vi "mod_Calculate Correction(Cont Zoom FFT).vi"(8 "error in (no error)":errorcluster, 9 "units":T3(ring)=enum."Watts", 10 "actual spectrum settings":T1={"center frequency"=-inf, "span"=-1.0, "resolution bandwidth"=-1.0, "window"=8, "spectral lines"=400, "%overlap"=0.0} {"%overlap" min=0.0 max=100.0 format="%.2f"; "window" items=["None ", "Hanning", "Hamming", "Blackman-Harris", "Exact Blackman", "Blackman", "Flat Top", "4 Term B-Harris ", "7 Term B-Harris", "Low Sidelobe"]; "resolution bandwidth" format="%.2p"; "center frequency" format="%.2p"; "span" format="%.2p"}, 11 "calibration array":T4(array[cluster]) {"array" format="%.2p"; "f2" format="%.2f"; "f1" format="%.2f"}) -> (0 "error out":errorcluster, 3 "correction":T2 {"spectrum correction"."correction factors" format="%.2f"; "spectrum correction"."df" format="%.2f"; "spectrum correction"."fo" format="%.2f"})   [LabVIEW 2020, in "niAMT.lvlib"]
doc: "Calculates a correction to compensate a spectrum for the amplitude response of signal conditioners and digitizers. Use your instrument drivers to determine the values you enter in the <B>calibration</B> cluster."
uses:
  <vilib>/addons/Modulation/niAMT.lvlib
  <vilib>/measure/masml.llb/ma_sml_CZ Spectrum Settings.ctl
  <vilib>/Analysis/1siggen.llb/Ramp Pattern by Samples.vi
  <vilib>/Analysis/NI_AALPro.lvlib
  <vilib>/Analysis/NI_AALBase.lvlib
  <vilib>/measure/NI_MAPro.lvlib
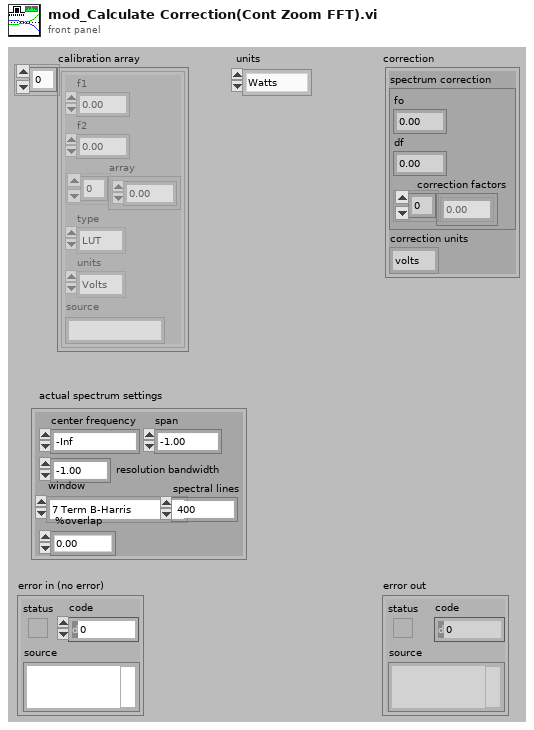
[diagram p1: front panel]
types:
  T1 = typedef "NI_MAPro.lvlib/ma_sml_CZ Spectrum Settings.ctl" = cluster{"center frequency":dbl, "span":dbl, "resolution bandwidth":dbl, "window":u16, "spectral lines":i32, "%overlap":dbl}
  T2 = cluster{"spectrum correction":cluster{"fo":dbl, "df":dbl, "correction factors":dbl[]}, "correction units":enum16{"volts", "watts", "dB"}}
  T3 = enum16{"Volts", "Watts", "dBm", "dBW", "dBV", "dBmV", "dBuV"}
  T4 = cluster{"f1":dbl, "f2":dbl, "array":sgl[], "type":enum16{"LUT", "polynomial"}, "units":enum16{"Volts", "Watts", "dBm", "dBW", "dBV", "dBmV", "dBuV"}, "source":string}[]
  T5 = cluster{cluster{dbl, dbl, dbl[]}, "correction units":enum16{"volts", "watts", "dB"}}
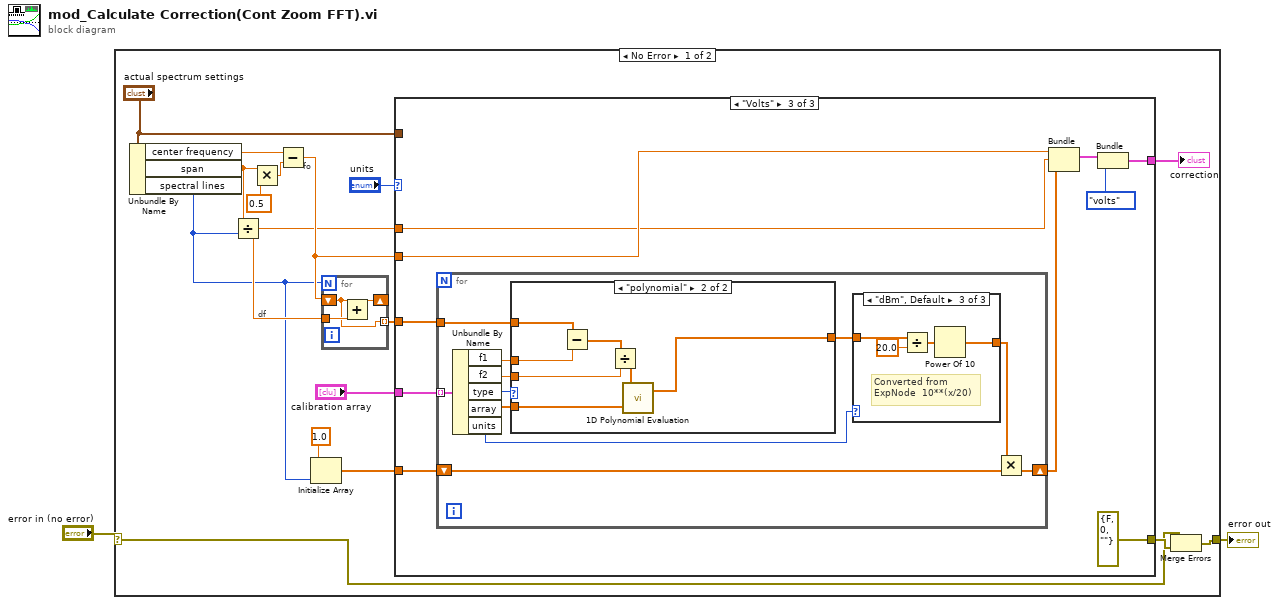
[diagram p0: block diagram]
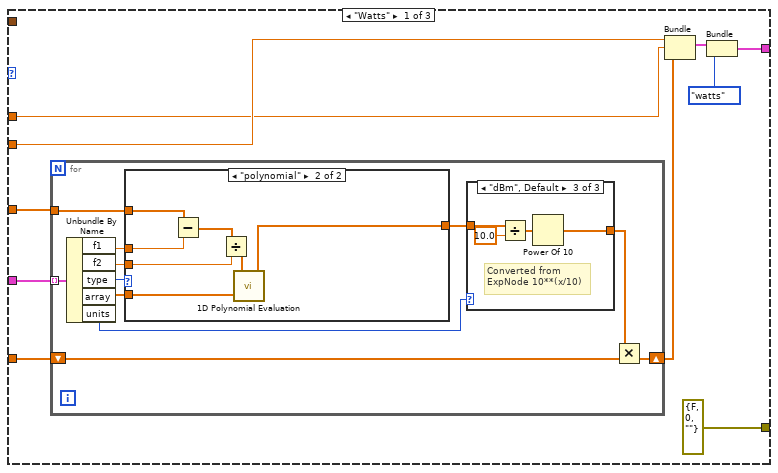
[diagram p2: hidden frame]
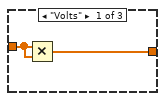
[diagram p3: hidden frame]
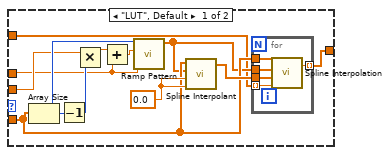
[diagram p5: hidden frame]
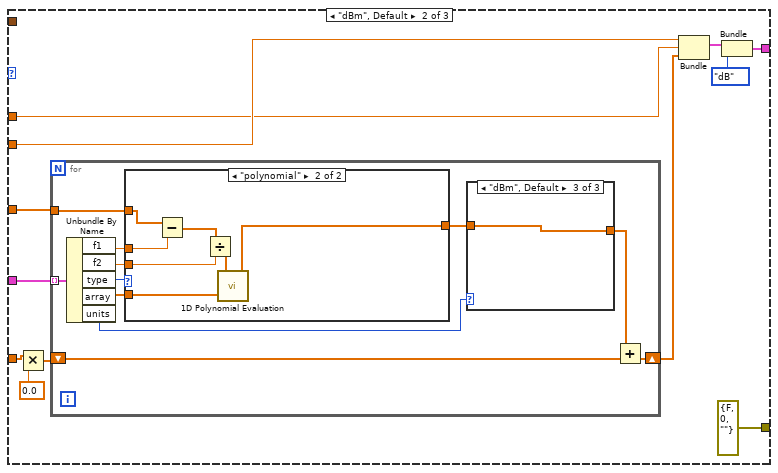
[diagram p6: hidden frame]
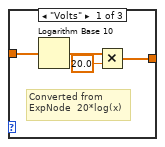
[diagram p7: hidden frame]
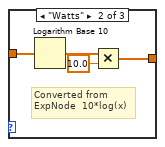
[diagram p8: hidden frame]
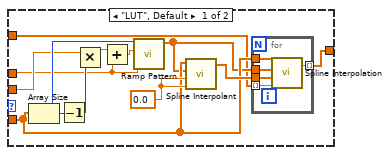
[diagram p9: hidden frame]
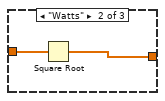
[diagram p11: hidden frame]
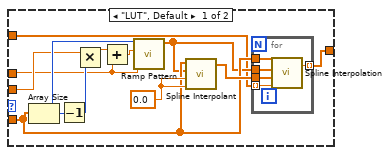
[diagram p12: hidden frame]
diagram:
  n1 = case shown="No Error" "error in (no error)" {
    selector: "error in (no error)" -> [w3 w183]
    tunnel: [w4 w183] -> w1
    frame No Error {
      # "df"
      # "fo"
      n2 = Unbundle By Name("actual spectrum settings") -> ("center frequency"=w15:dbl, "span"=w12:dbl, "spectral lines"=w7:i32)
      n3 = Divide(x=w12, y=w7) -> (x/y=w10:dbl)
      n4 = Multiply(x=w12, y=0.5) -> (x*y=w14:dbl)
      n5 = Subtract(x=w15, y=w14) -> (x-y=w11:dbl)
      n6 = Initialize Array(1.0, w7) -> (w17:dbl[])
      n7 = for {
        N: w7 -> [_]
        shift-right: [w181] -> _
        shift-left: w11 -> [w180]
        tunnel: w10 -> [w182]
        tunnel: [w180] -> w18 mode=indexing
        n8 = Add(x=w180, y=w182) -> (x+y=w181:dbl)
      }
      n9 = case shown="\"Volts\"" "units" {
        tunnel: "calibration array" -> [w29 w83 w137]
        tunnel: "actual spectrum settings" -> [_ _ _]
        tunnel: w18 -> [w28 w82 w136]
        tunnel: w17 -> [w26 w80 w134]
        tunnel: [errorcluster {"status"=FALSE, "code"=0, "source"=""} ("error IO") errorcluster {"status"=FALSE, "code"=0, "source"=""} ("error IO") errorcluster {"status"=FALSE, "code"=0, "source"=""} ("error IO")] -> w5
        tunnel: w11 -> [w25 w79 w133]
        tunnel: w10 -> [w24 w78 w132]
        tunnel: [w21 w75 w129] -> w8
        frame "Watts" {
          n10 = for {
            tunnel: w29 -> [w38] mode=indexing
            tunnel: w28 -> [w39]
            shift-right: [w30] -> w23
            shift-left: w26 -> [w32]
            n11 = Unbundle By Name(w38) -> ("f1"=w34:dbl, "f2"=w33:dbl, "type"=w40:enum16{"LUT", "polynomial"}, "array"=w37:sgl[], "units"=w36:T3)
            n12 = case shown="\"polynomial\"" w40 {
              tunnel: w39 -> [w49 w66]
              tunnel: w37 -> [w51 w68]
              tunnel: [w48 w65] -> w35
              tunnel: w34 -> [w53 w67]
              tunnel: w33 -> [w57 w69]
              frame "LUT", Default {
                w59 = 0.0 ("initial boundary")
                n13 = Array Size(array=w51) -> (size(s)=w58:i32)
                n14 = Decrement(x=w58) -> (x-1=w56:i32)
                n15 = Multiply(x=w57, y=w56) -> (x*y=w54:dbl)
                n16 = Add(x=w54, y=w53) -> (x+y=w55:dbl)
                n17 = call-poly <vilib>:"Ramp Pattern.vi"("start"=w53, "end"=w55, "samples"=w58) -> ("Ramp Pattern"=w50:dbl[])  [unwired: 7 in, 1 out]
                n18 = call <vilib>:"Spline Interpolant.vi"("final boundary"=w59, "initial boundary"=w59, "X"=w50, "Y"=w51) -> ("Interpolant"=w52:dbl[])  [unwired: 1 out]
                n19 = for {
                  tunnel: w52 -> [w64]
                  tunnel: w51 -> [w63]
                  tunnel: w50 -> [w62]
                  tunnel: w49 -> [w61] mode=indexing
                  tunnel: [w60] -> w48 mode=indexing
                  n20 = call <vilib>:"Spline Interpolation.vi"("x value"=w61, "Interpolant"=w64, "X"=w62, "Y"=w63) -> ("interpolation value"=w60:dbl)  [unwired: 1 out]
                }
              }
              frame "polynomial" {
                n21 = Subtract(x=w66, y=w67) -> (x-y=w71:dbl[])
                n22 = Divide(x=w71, y=w69) -> (x/y=w70:dbl[])
                n23 = call <vilib>:"1D Polynomial Evaluation.vi"("Coefficients: a"=w68, "X"=w70) -> ("Y"=w65:dbl[])  [unwired: 1 out]
              }
            }
            n24 = case shown="\"dBm\", Default" w36 {
              tunnel: w35 -> [w41 w43 w45]
              tunnel: [w42 w43 w44] -> w31
              frame "Volts" {
                n25 = Multiply(x=w41, y=w41) -> (x*y=w42:dbl[])
              }
              frame "Watts" {
              }
              frame "dBm", Default {
                # "Converted from\nExpNode 10**(x/10)"
                n26 = Divide(x=w45, y=10.0) -> (x/y=w47:dbl[])
                n27 = Power Of 10(x=w47) -> (10^x=w44:dbl[])
              }
            }
            n28 = Multiply(x=w31, y=w32) -> (x*y=w30:dbl[])
          }
          n29 = Bundle(w25, w24, w23) -> (w22:cluster{dbl, dbl, dbl[]})  [unwired: 1 out]
          n30 = Bundle(w22, "correction units"=enum16{"volts", "watts", "dB"}."watts") -> (w21:T5)  [unwired: 1 out]
        }
        frame "dBm", Default {
          n31 = Multiply(x=w80, y=0.0) -> (x*y=w74:dbl[])
          n32 = for {
            tunnel: w83 -> [w92] mode=indexing
            tunnel: w82 -> [w93]
            shift-right: [w84] -> w77
            shift-left: w74 -> [w86]
            n33 = Unbundle By Name(w92) -> ("f1"=w88:dbl, "f2"=w87:dbl, "type"=w94:enum16{"LUT", "polynomial"}, "array"=w91:sgl[], "units"=w90:T3)
            n34 = case shown="\"polynomial\"" w94 {
              tunnel: w93 -> [w105 w127]
              tunnel: w91 -> [w107 w126]
              tunnel: [w104 w125] -> w89
              tunnel: w88 -> [w109 w123]
              tunnel: w87 -> [w113 w121]
              frame "LUT", Default {
                w115 = 0.0 ("initial boundary")
                n35 = Array Size(array=w107) -> (size(s)=w114:i32)
                n36 = Decrement(x=w114) -> (x-1=w112:i32)
                n37 = Multiply(x=w113, y=w112) -> (x*y=w110:dbl)
                n38 = Add(x=w110, y=w109) -> (x+y=w111:dbl)
                n39 = call-poly <vilib>:"Ramp Pattern.vi"("start"=w109, "end"=w111, "samples"=w114) -> ("Ramp Pattern"=w106:dbl[])  [unwired: 7 in, 1 out]
                n40 = call <vilib>:"Spline Interpolant.vi"("final boundary"=w115, "initial boundary"=w115, "X"=w106, "Y"=w107) -> ("Interpolant"=w108:dbl[])  [unwired: 1 out]
                n41 = for {
                  tunnel: w108 -> [w120]
                  tunnel: w107 -> [w119]
                  tunnel: w106 -> [w118]
                  tunnel: w105 -> [w117] mode=indexing
                  tunnel: [w116] -> w104 mode=indexing
                  n42 = call <vilib>:"Spline Interpolation.vi"("x value"=w117, "Interpolant"=w120, "X"=w118, "Y"=w119) -> ("interpolation value"=w116:dbl)  [unwired: 1 out]
                }
              }
              frame "polynomial" {
                n43 = Subtract(x=w127, y=w123) -> (x-y=w124:dbl[])
                n44 = Divide(x=w124, y=w121) -> (x/y=w122:dbl[])
                n45 = call <vilib>:"1D Polynomial Evaluation.vi"("Coefficients: a"=w126, "X"=w122) -> ("Y"=w125:dbl[])  [unwired: 1 out]
              }
            }
            n46 = case shown="\"dBm\", Default" w90 {
              tunnel: w89 -> [w96 w100 w103]
              tunnel: [w95 w99 w103] -> w85
              frame "Volts" {
                # "Converted from\nExpNode \t20*log(x)"
                n47 = Logarithm Base 10(1:w96) -> (0:w97:dbl[])
                n48 = Multiply(x=w97, y=20.0) -> (x*y=w95:dbl[])
              }
              frame "Watts" {
                # "Converted from\nExpNode \t10*log(x)"
                n49 = Logarithm Base 10(1:w100) -> (0:w101:dbl[])
                n50 = Multiply(x=w101, y=10.0) -> (x*y=w99:dbl[])
              }
              frame "dBm", Default {
              }
            }
            n51 = Add(x=w85, y=w86) -> (x+y=w84:dbl[])
          }
          n52 = Bundle(w79, w78, w77) -> (w76:cluster{dbl, dbl, dbl[]})  [unwired: 1 out]
          n53 = Bundle(w76, "correction units"=enum16{"volts", "watts", "dB"}."dB") -> (w75:T5)  [unwired: 1 out]
        }
        frame "Volts" {
          n54 = for {
            tunnel: w137 -> [w146] mode=indexing
            tunnel: w136 -> [w147]
            shift-right: [w138] -> w131
            shift-left: w134 -> [w140]
            n55 = Unbundle By Name(w146) -> ("f1"=w142:dbl, "f2"=w141:dbl, "type"=w148:enum16{"LUT", "polynomial"}, "array"=w145:sgl[], "units"=w144:T3)
            n56 = case shown="\"polynomial\"" w148 {
              tunnel: w147 -> [w157 w174]
              tunnel: w145 -> [w159 w173]
              tunnel: [w156 w179] -> w143
              tunnel: w142 -> [w161 w175]
              tunnel: w141 -> [w165 w176]
              frame "LUT", Default {
                w167 = 0.0 ("initial boundary")
                n57 = Array Size(array=w159) -> (size(s)=w166:i32)
                n58 = Decrement(x=w166) -> (x-1=w164:i32)
                n59 = Multiply(x=w165, y=w164) -> (x*y=w162:dbl)
                n60 = Add(x=w162, y=w161) -> (x+y=w163:dbl)
                n61 = call-poly <vilib>:"Ramp Pattern.vi"("start"=w161, "end"=w163, "samples"=w166) -> ("Ramp Pattern"=w158:dbl[])  [unwired: 7 in, 1 out]
                n62 = call <vilib>:"Spline Interpolant.vi"("final boundary"=w167, "initial boundary"=w167, "X"=w158, "Y"=w159) -> ("Interpolant"=w160:dbl[])  [unwired: 1 out]
                n63 = for {
                  tunnel: w160 -> [w172]
                  tunnel: w159 -> [w171]
                  tunnel: w158 -> [w170]
                  tunnel: w157 -> [w169] mode=indexing
                  tunnel: [w168] -> w156 mode=indexing
                  n64 = call <vilib>:"Spline Interpolation.vi"("x value"=w169, "Interpolant"=w172, "X"=w170, "Y"=w171) -> ("interpolation value"=w168:dbl)  [unwired: 1 out]
                }
              }
              frame "polynomial" {
                n65 = Subtract(x=w174, y=w175) -> (x-y=w178:dbl[])
                n66 = Divide(x=w178, y=w176) -> (x/y=w177:dbl[])
                n67 = call <vilib>:"1D Polynomial Evaluation.vi"("Coefficients: a"=w173, "X"=w177) -> ("Y"=w179:dbl[])  [unwired: 1 out]
              }
            }
            n68 = case shown="\"dBm\", Default" w144 {
              tunnel: w143 -> [w149 w151 w153]
              tunnel: [w149 w150 w152] -> w139
              frame "Volts" {
              }
              frame "Watts" {
                n69 = Square Root(x=w151) -> (sqrt(x)=w150:dbl[])
              }
              frame "dBm", Default {
                # "Converted from\nExpNode \t10**(x/20)"
                n70 = Divide(x=w153, y=20.0) -> (x/y=w154:dbl[])
                n71 = Power Of 10(x=w154) -> (10^x=w152:dbl[])
              }
            }
            n72 = Multiply(x=w139, y=w140) -> (x*y=w138:dbl[])
          }
          n73 = Bundle(w133, w132, w131) -> (w130:cluster{dbl, dbl, dbl[]})  [unwired: 1 out]
          n74 = Bundle(w130, "correction units"=enum16{"volts", "watts", "dB"}."volts") -> (w129:T5)  [unwired: 1 out]
        }
      }
      "correction" <- w8
      n75 = Merge Errors(w3, w5) -> (w4:errorcluster)
    }
    frame Error {
    }
  }
  "error out" <- w1
